vi "Help - Lookup CMH Path.vi"(1 "Main CMH File":string) -> (0 "Compiled CMH Path":path)   [LabVIEW 2016, in "UDP-Custom-Device System Explorer.lvlib"]
uses:
  UDP-Custom-Device System Explorer.lvlib
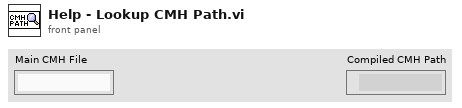
[diagram p1: front panel]
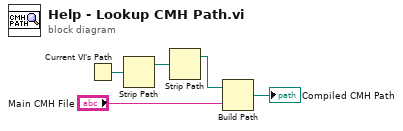
[diagram p0: block diagram]
diagram:
  n1 = Current VI's Path() -> (path=w5:path)
  n2 = Strip Path(path=w5) -> (stripped path=w4:path)  [unwired: 1 out]
  n3 = Strip Path(path=w4) -> (stripped path=w3:path)  [unwired: 1 out]
  n4 = Build Path(base path=w3, name or relative path="Main CMH File") -> (appended path=→"Compiled CMH Path":path)
